vi "SPD.Set Single Point Meas Grid.vi"(7 "Temprature":dbl, 8 "Error In":errorcluster, 9 "HV_bias":dbl, 10 "Strobe_code":dbl, 11 "SPD.Stand Ctrl in":T1={"spdDeviceSession"={"spdRef"=0, "connected"=FALSE, "spdName"="", "specification"={"diod case"=enum."default", "type"=enum."Unknown", "frequency"=enum."Unknown"}, "hidSPD.Controller"={"TSet"=0.0, "HV_bias"=0.0, "DDS_stb_code"=0}, "hidSPD.Sturtup Values"={"TSet"=0.0, "HV_bias"=0.0, "DDS_stb_code"=0}}, "DevBSession"={"DevBRef"="", "connected"=FALSE}, "FreqCSession"={"FreqCRef"="", "timeout"=0.0, "Gate"=0.0, "connected"=FALSE}, "8164BSession"={"Connection ID"=refnum, "Connected"=FALSE, "Info"="", "Slots Info"=[]}, "LeCroySession"={"LeCroySession"="", "connected"=FALSE}, "Events"={"DCRTest"=refnum, "Stop"=refnum}, "configFile"={"configFile ref"=refnum, "configFile path"=path "", "equipmentFile ref"=refnum}, "SPD.Meas Grid"={"DateTime"="", "DT"=[], "Insensitivity"=[], "Temprature"=[], "Stb_code"=[], "HV_Bias"=[]}, "SPD.Queues"={"state queue"=refnum}, "Console"=refnum} {"spdDeviceSession"."hidSPD.Sturtup Values"."HV_bias" format="%#_6p, V"; "spdDeviceSession"."hidSPD.Sturtup Values"."TSet" format="%#_6p, DegC"; "spdDeviceSession"."hidSPD.Controller"."HV_bias" format="%#_6p, V"; "spdDeviceSession"."hidSPD.Controller"."TSet" format="%#_6p, DegC"}) -> (0 "Error Out":errorcluster, 3 "SPD.Stand Ctrl out":T1={"spdDeviceSession"={"spdRef"=0, "connected"=FALSE, "spdName"="", "specification"={"diod case"=enum."default", "type"=enum."Unknown", "frequency"=enum."Unknown"}, "hidSPD.Controller"={"TSet"=0.0, "HV_bias"=0.0, "DDS_stb_code"=0}, "hidSPD.Sturtup Values"={"TSet"=0.0, "HV_bias"=0.0, "DDS_stb_code"=0}}, "DevBSession"={"DevBRef"="", "connected"=FALSE}, "FreqCSession"={"FreqCRef"="", "timeout"=0.0, "Gate"=0.0, "connected"=FALSE}, "8164BSession"={"Connection ID"=refnum, "Connected"=FALSE, "Info"="", "Slots Info"=[]}, "LeCroySession"={"LeCroySession"="", "connected"=FALSE}, "Events"={"DCRTest"=refnum, "Stop"=refnum}, "configFile"={"configFile ref"=refnum, "configFile path"=path "", "equipmentFile ref"=refnum}, "SPD.Meas Grid"={"DateTime"="", "DT"=[], "Insensitivity"=[], "Temprature"=[], "Stb_code"=[], "HV_Bias"=[]}, "SPD.Queues"={"state queue"=refnum}, "Console"=refnum} {"spdDeviceSession"."hidSPD.Sturtup Values"."HV_bias" format="%#_6p, V"; "spdDeviceSession"."hidSPD.Sturtup Values"."TSet" format="%#_6p, DegC"; "spdDeviceSession"."hidSPD.Controller"."HV_bias" format="%#_6p, V"; "spdDeviceSession"."hidSPD.Controller"."TSet" format="%#_6p, DegC"})   [LabVIEW 2018]
uses:
  Instruments/KC705 DevBoard/typedefs/DevB.Session.ctl
  Instruments/KeySight 53230A/typedefs/FreqC.Session.ctl
  Instruments/KeySight 8164B/KeySight 8164B LAN InstrLib/typedefs/KeySight 8164B control.ctl
  Instruments/KeySight 8164B/KeySight 8164B LAN InstrLib.lvlib
  Instruments/LeCroy SDA830/typedefs/LeCroy.Session.ctl
  typedefs/SPD.Events.ctl
  <vilib>/Utility/config.llb/Config Data RefNum.ctl
  <vilib>/Utility/config.llb/NI_LVConfig.lvlib
  typedefs/SPD.Meas Grid.ctl
  typedefs/SPD.Stand Ctrl.ctl
  typedefs/SPD.Stand state.ctl
  typedefs/SPD.Queues.ctl
  ConfigFile/SPD.Config File ctrl.ctl
  Instruments/SPD HID Interface/hidSPDLibForLabView/LibVIs/hidSPD Controls/hidSPD Controller.ctl
  Instruments/SPD HID Interface/hidSPDLibForLabView/hidSPDLibForLabView.lvlib
  Instruments/SPD HID Interface/hidSPDLibForLabView/LibVIs/hidSPD Controls/hidSPD Device Session.ctl
  Instruments/SPD HID Interface/hidSPDLibForLabView/LibVIs/hidSPD Controls/hidSPD SPD Type.ctl
  Instruments/SPD HID Interface/hidSPDLibForLabView/LibVIs/hidSPD Controls/hidSPD SPD Diod Case.ctl
  Instruments/SPD HID Interface/hidSPDLibForLabView/LibVIs/hidSPD Controls/hidSPD.STB Frequency.ctl
  Instruments/SPD HID Interface/hidSPDLibForLabView/LibVIs/hidSPD Controls/hidSPD.SPD specification.ctl
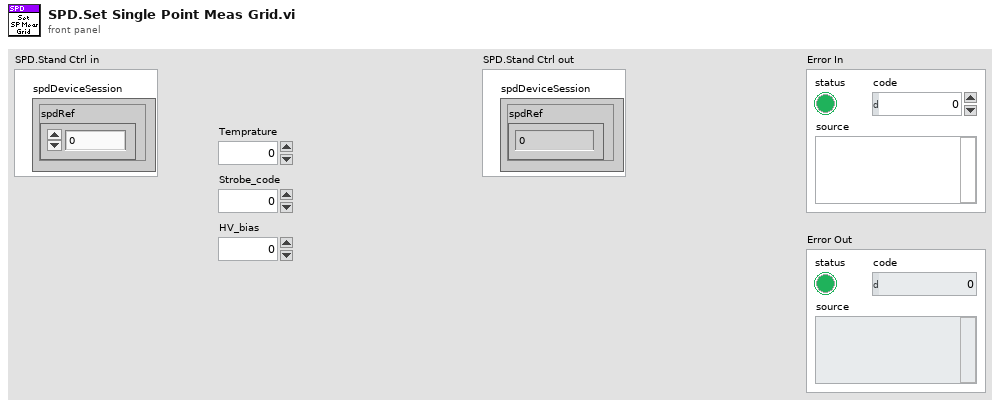
[diagram p1: front panel]
types:
  T1 = typedef "SPD.Stand Ctrl.ctl" = cluster{"spdDeviceSession":T2, "DevBSession":T8, "FreqCSession":T9, "8164BSession":T10, "LeCroySession":T11, "Events":T12, "configFile":T13, "SPD.Meas Grid":T15, "SPD.Queues":T16, "Console":refnum<vi>}
  T2 = typedef "hidSPDLibForLabView.lvlib/hidSPD Device Session.ctl" = cluster{"spdRef":u64, "connected":bool, "spdName":string, "specification":T3, "hidSPD.Controller":T7, "hidSPD.Sturtup Values":T7}
  T3 = typedef "hidSPDLibForLabView.lvlib/hidSPD.SPD specification.ctl" = cluster{"diod case":T4, "type":T5, "frequency":T6}
  T4 = typedef "hidSPDLibForLabView.lvlib/hidSPD SPD Diod Case.ctl" = enum16{"Unknown", "default", "butterfly"}
  T5 = typedef "hidSPDLibForLabView.lvlib/hidSPD SPD Type.ctl" = enum16{"Unknown", "Free Run", "Gate"}
  T6 = typedef "hidSPDLibForLabView.lvlib/hidSPD.STB Frequency.ctl" = enum16{"Unknown", "312", "1250"}
  T7 = typedef "hidSPDLibForLabView.lvlib/hidSPD Controller.ctl" = cluster{"TSet":sgl, "HV_bias":sgl, "DDS_stb_code":u16}
  T8 = typedef "DevB.Session.ctl" = cluster{"DevBRef":refnum<visa-resource-name>, "connected":bool}
  T9 = typedef "FreqC.Session.ctl" = cluster{"FreqCRef":refnum<visa-resource-name>, "timeout":dbl, "Gate":dbl, "connected":bool}
  T10 = typedef "KeySight 8164B LAN InstrLib.lvlib/KeySight 8164B control.ctl" = cluster{"Connection ID":refnum<k5>, "Connected":bool, "Info":string, "Slots Info":string[]}
  T11 = typedef "LeCroy.Session.ctl" = cluster{"LeCroySession":refnum<visa-resource-name>, "connected":bool}
  T12 = typedef "SPD.Events.ctl" = cluster{"DCRTest":refnum<user-event>, "Stop":refnum<user-event>}
  T13 = typedef "SPD.Config File ctrl.ctl" = cluster{"configFile ref":T14, "configFile path":path, "equipmentFile ref":T14}
  T14 = typedef "NI_LVConfig.lvlib/Config Data RefNum.ctl" = refnum<k1>
  T15 = typedef "SPD.Meas Grid.ctl" = cluster{"DateTime":string, "DT":dbl[], "Insensitivity":dbl[], "Temprature":dbl[], "Stb_code":dbl[], "HV_Bias":dbl[][][][]}
  T16 = typedef "SPD.Queues.ctl" = cluster{"state queue":refnum<queue>}
  T17 = typedef "hidSPDLibForLabView.lvlib/hidSPD SPD Type.ctl" = enum16{"Unknown", "Free Run", "Gate_312", "Gate_1250"}
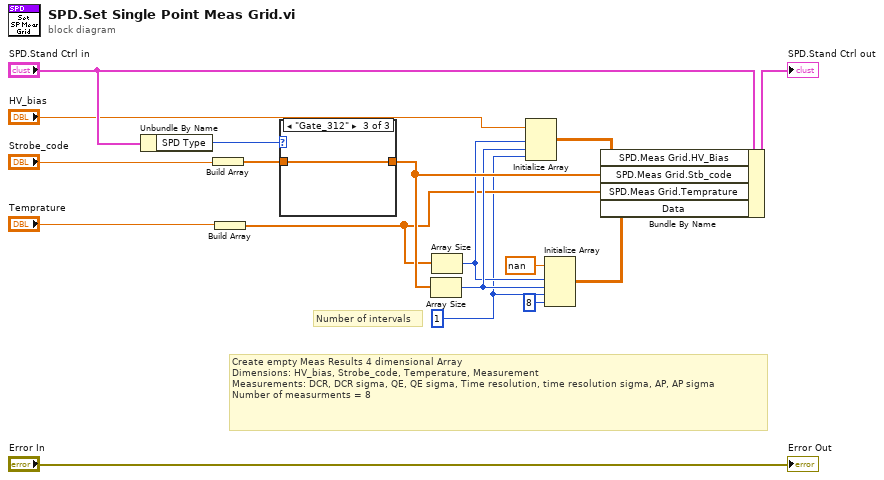
[diagram p0: block diagram]
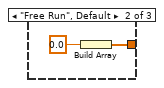
[diagram p3: hidden frame]
diagram:
  w1 = 1 ("dimension size")
  # "Number of intervals"
  # "Create empty Meas Results 4 dimensional Array\nDimensions: HV_bias, Strobe_code, Temperature, Measurement\nMeasurements: DCR, DCR sigma, QE, QE sigma, Time resolution, time resolution sigma, AP, AP sigma\nNumber of measurments = 8"
  n1 = Unbundle By Name("SPD.Stand Ctrl in") -> ("SPD Type"=w7:T17)
  n2 = Build Array("Strobe_code") -> (w3:dbl[])
  n3 = Build Array("Temprature") -> (w5:dbl[])
  n4 = case shown="\"Gate_312\"" w7 {
    tunnel: [_ w18 w20] -> w15
    tunnel: w3 -> [_ _ w20]
    frame "Unknown" {
    }
    frame "Free Run", Default {
      n5 = Build Array(0.0) -> (w18:dbl[])
    }
    frame "Gate_312" {
    }
  }
  n6 = Array Size(array=w15) -> (size(s)=w11:i32)
  n7 = Array Size(array=w5) -> (size(s)=w9:i32)
  n8 = Initialize Array("HV_bias", w9, w11, w1) -> (w10:dbl[][][])
  n9 = Initialize Array(nan ("element"), w9, w11, w1, 8 ("dimension size")) -> (w12:dbl[][][][])
  n10 = Bundle By Name(cluster="SPD.Stand Ctrl in", "SPD.Meas Grid.HV_Bias"=w10, "SPD.Meas Grid.Stb_code"=w15, "SPD.Meas Grid.Temprature"=w5, "Data"=w12) -> (→"SPD.Stand Ctrl out":T1)
  "Error Out" <- "Error In"
